vi "GetDxAndDyforhaverine.vi"(8 "distance (dm)":dbl, 10 "polar angle":dbl, 11 "compassHeading":dbl) -> (0 "dx":dbl, 3 "dy":dbl)   [LabVIEW 2011]
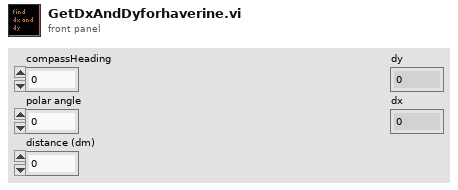
[diagram p1: front panel]
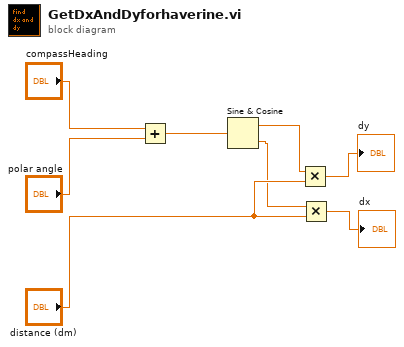
[diagram p0: block diagram]
diagram:
  n1 = Add(x="compassHeading", y="polar angle") -> (x+y=w6:dbl)
  n2 = Sine & Cosine(0:w6) -> (1:w3:dbl, 2:w4:dbl)
  n3 = Multiply(x=w3, y="distance (dm)") -> (x*y=→"dy":dbl)
  n4 = Multiply(x=w4, y="distance (dm)") -> (x*y=→"dx":dbl)
